vi "weight_experimental2.vi"(9 "IIR Filter Cluster":T1={"filter structure"=enum."IIR 2nd Order", "Reverse Coefficients"=[-0.8648355985677569, 0.0, -1.8688121229267716, 0.9029397901016704, -1.8196275590015545, 0.847351865339388, -1.7873550514945042, 0.8113653291402647, -1.7646245178602125, 0.7862391997716377, -1.7486001722944886, 0.7686314023380645, -1.7316927626267011, 0.7501448296370037, -1.737874982086305, 0.7568937398228854], "Forward Coefficients"=[0.0742867069172382, 0.0742867069172382, 0.0, 0.005985276674302437, 0.011970553348604874, 0.005985276674302437, 0.00581901644640044, 0.01163803289280088, 0.00581901644640044, 0.005710698277145051, 0.011421396554290102, 0.005710698277145051, 0.005634756015992636, 0.011269512031985273, 0.005634756015992636, 0.005581386206513606, 0.011162772413027213, 0.005581386206513606, 0.0055252205885281845, 0.011050441177056369, 0.0055252205885281845, 0.00554574059897006, 0.01109148119794012, 0.00554574059897006]}, 10 "N_points":i32=4200, 11 "PV weight":dbl caption="g" format="%#.0f") -> (1 "Q3":dbl caption="mg/s" format="%#.0f", 2 "Q 1":dbl caption="mg/s" format="%#.0f", 3 "Weight 1":dbl caption="g" format="%#.0f", 5 "This VI":refnum<vi>)   [LabVIEW 2019]
uses:
  <vilib>/Analysis/baseanly.llb/Mean (DBL).vi
  <vilib>/Analysis/baseanly.llb/IIR Cascade Filter (DBL).vi
  <vilib>/Analysis/NI_AALBase.lvlib
panel:
  in  "Tab Control":T2(tab)
  out "dM 3":dbl caption="g" format="%#.0f"
  out "dM 1":dbl caption="g" format="%#.0f"
  out "variance":dbl format="%0.2f"
  out "standard deviation":dbl format="%0.2f"
  in  "Tare":dbl caption="g" format="%#.0f"
  in  "<0>":bool
  in  "<вес>":bool
  in  "k":dbl=1.0 caption="g" format="%#.3f"
  in  "Вес":dbl caption="g" format="%#.0f"
  # "Усреднение за 1 мин"
  # "(расход)"
  # "Усреднение за 3 мин"
  # "(расход)"
  # "Вес тары\n(полностью очистить бункер от продукта\nи запомнить PV weight или ввести вручную)."
  # "Вес тары\n(ввести фактический вес без учета тары\nили ввести k вручную)"
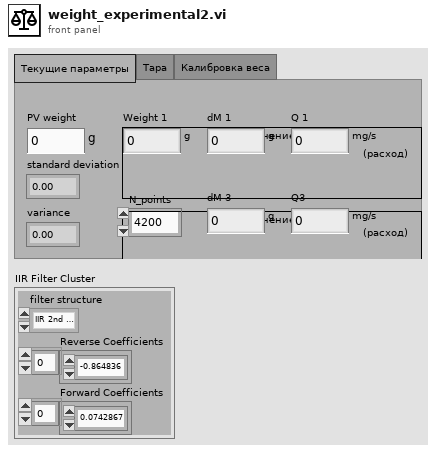
[diagram p1: front panel]
types:
  T1 = cluster{"filter structure":enum32{"IIR 2nd Order", "IIR 4th Order"}, "Reverse Coefficients":dbl[], "Forward Coefficients":dbl[]}
  T2 = enum32{"Текущие параметры", "Тара", "Калибровка веса"}
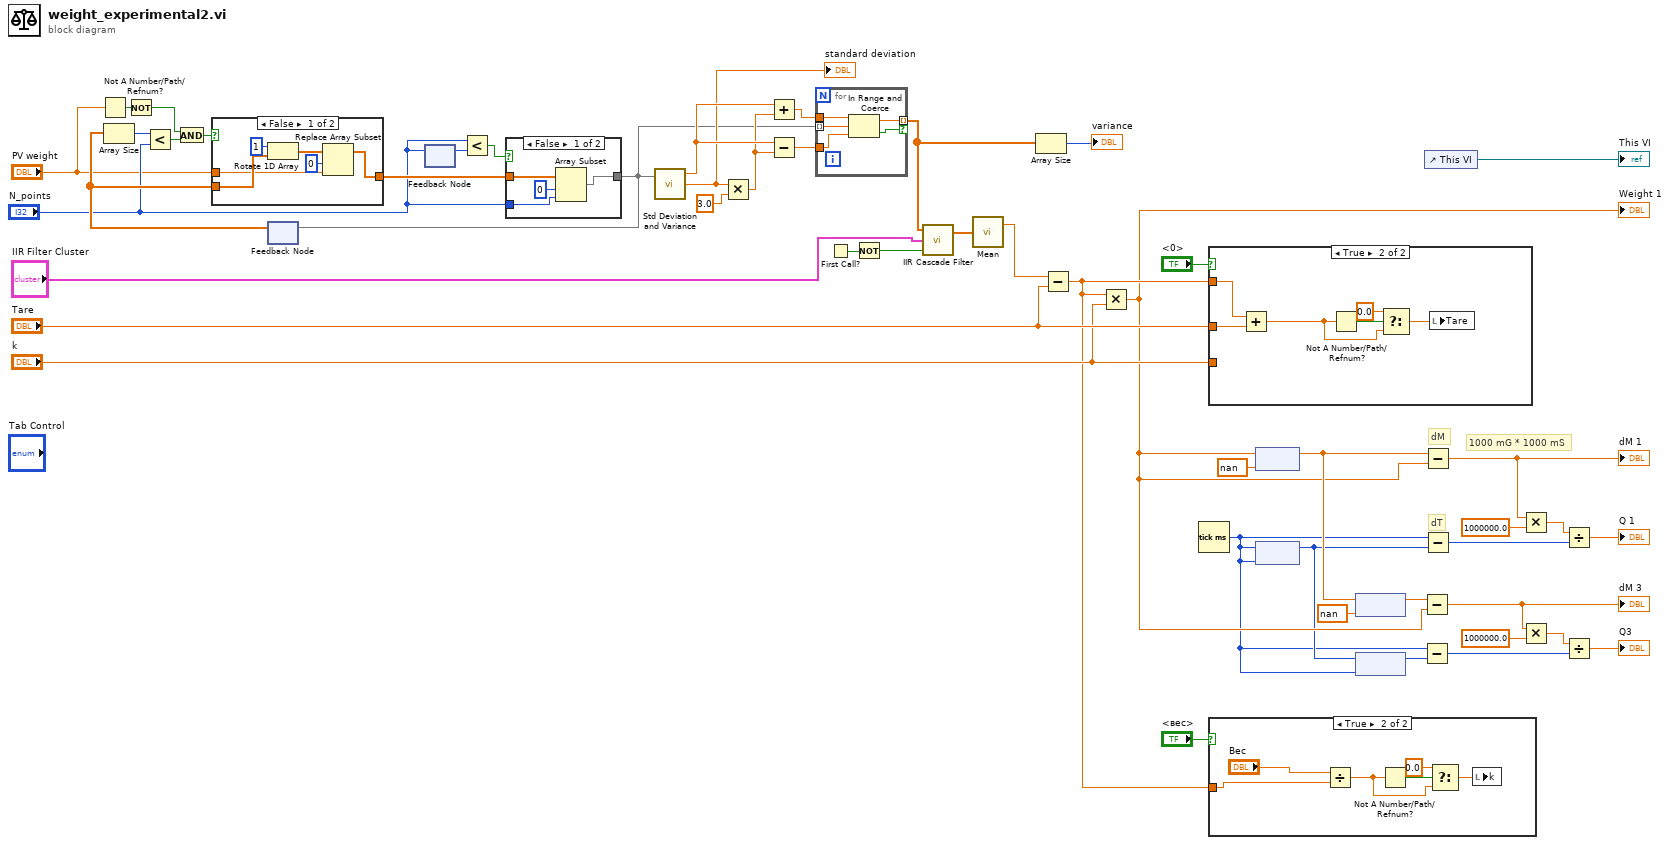
[diagram p0: block diagram]
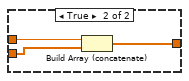
[diagram p3: hidden frame]
diagram:
  # "1000 mG * 1000 mS"
  # "dM"
  # "dT"
  n1 = Not A Number/Path/Refnum?(number/path/refnum="PV weight") -> (NaN/Path/Refnum?=w14:bool)
  n2 = Not(x=w14) -> (.not. x?=w13:bool)
  n3 = feedback #1() -> (w17:dbl[])  [unwired: 1 in]
  n4 = Array Size(array=w17) -> (size(s)=w18:i32)
  n5 = Less?(x=w18, y="N_points") -> (x < y?=w16:bool)
  n6 = And(x=w13, y=w16) -> (x .and. y?=w15:bool)
  n7 = case shown="False" w15 {
    tunnel: [w50 w57] -> w12
    tunnel: "PV weight" -> [w51 w58]
    tunnel: w17 -> [w52 w56]
    frame False {
      n8 = Rotate 1D Array(1:w52, 2:1 ("n")) -> (0:w54:dbl[])
      n9 = Replace Array Subset(array=w54, new element=w51, index=0) -> (w50:dbl[])
    }
    frame True {
      n10 = Build Array (concatenate)(w58, w56) -> (w57:dbl[])
    }
  }
  n11 = feedback #2() -> (w10:i32)  [unwired: 1 in]
  n12 = feedback-in #2("N_points") -> ()
  n13 = Less?(x="N_points", y=w10) -> (x < y?=w9:bool)
  n14 = case shown="False" w9 {
    tunnel: [w61 w63] -> w8
    tunnel: w12 -> [w62 w63]
    tunnel: "N_points" -> [w59 _]
    frame False {
      n15 = Array Subset(array=w62, index=0, length=w59) -> (w61:dbl[])
    }
    frame True {
    }
  }
  n16 = feedback-in #1(w8) -> ()
  n17 = call <vilib>:"Std Deviation and Variance.vi"("X"=w8) -> ("mean"=w25:dbl, "standard deviation"=w21:dbl)  [unwired: 1 in, 1 out]
  "standard deviation" <- w21
  n18 = Multiply(x=w21, y=3.0) -> (x*y=w19:dbl)
  n19 = Add(x=w25, y=w19) -> (x+y=w24:dbl)
  n20 = Subtract(x=w25, y=w19) -> (x-y=w23:dbl)
  n21 = for {
    tunnel: w8 -> [w66] mode=indexing
    tunnel: w24 -> [w68]
    tunnel: w23 -> [w67]
    tunnel: [w65] -> w3 mode=indexing if=w64
    n22 = In Range and Coerce(upper limit=w68, x=w66, lower limit=w67) -> (coerced(x)=w65:dbl, In Range?=w64:bool)
  }
  n23 = First Call?() -> (First Call?: T/F=w7:bool)
  n24 = Not(x=w7) -> (.not. x?=w6:bool)
  n25 = call-poly <vilib>:"IIR Cascade Filter.vi"("init/cont (init:F)"=w6, "IIR Filter Cluster"="IIR Filter Cluster", "X"=w3) -> ("Filtered X"=w2:dbl[])  [unwired: 1 out]
  n26 = call-poly <vilib>:"Mean.vi"("X"=w2) -> ("mean"=w1:dbl)  [unwired: 1 out]
  n27 = Array Size(array=w3) -> (size(s)=→"variance":i32)
  n28 = Subtract(x=w1, y="Tare") -> (x-y=w36:dbl)
  n29 = Multiply(x=w36, y="k") -> (x*y=w34:dbl)
  "Weight 1" <- w34
  n30 = Tick Count (ms)() -> (millisecond timer value=w31:u32)
  n31 = case shown="True" "<0>" {
    tunnel: "Tare" -> [_ w71]
    tunnel: w36 -> [_ w70]
    tunnel: "k" -> [_ _]
    frame False {
    }
    frame True {
      n32 = Add(x=w70, y=w71) -> (x+y=w69:dbl)
      n33 = Not A Number/Path/Refnum?(number/path/refnum=w69) -> (NaN/Path/Refnum?=w74:bool)
      n34 = Select(t=0.0 ("y"), s=w74, f=w69) -> (s? t:f=w72:dbl)
      n35 = local write "Tare"(w72) -> ()
    }
  }
  n36 = case shown="True" "<вес>" {
    tunnel: w36 -> [_ w75]
    frame False {
    }
    frame True {
      n37 = Divide(x="Вес", y=w75) -> (x/y=w78:dbl)
      n38 = Not A Number/Path/Refnum?(number/path/refnum=w78) -> (NaN/Path/Refnum?=w80:bool)
      n39 = Select(t=0.0 ("y"), s=w80, f=w78) -> (s? t:f=w77:dbl)
      n40 = local write "k"(w77) -> ()
    }
  }
  n41 = feedback #3(nan) -> (w45:dbl)
  n42 = feedback-in #3(w34) -> ()
  n43 = feedback #4(w31) -> (w33:u32)
  n44 = feedback-in #4(w31) -> ()
  n45 = feedback #5(nan) -> (w46:dbl)
  n46 = feedback-in #5(w45) -> ()
  n47 = feedback #6(w31) -> (w32:u32)
  n48 = feedback-in #6(w33) -> ()
  n49 = Subtract(x=w46, y=w34) -> (x-y=w27:dbl)
  "dM 3" <- w27
  n50 = Subtract(x=w31, y=w32) -> (x-y=w28:u32)
  n51 = Subtract(x=w45, y=w34) -> (x-y=w40:dbl)
  "dM 1" <- w40
  n52 = Subtract(x=w31, y=w33) -> (x-y=w38:u32)
  n53 = control-ref of="This VI"() -> (→"This VI":refnum<vi>)
  n54 = Multiply(x=w40, y=1000000.0) -> (x*y=w39:dbl)
  n55 = Multiply(x=w27, y=1000000.0) -> (x*y=w30:dbl)
  n56 = Divide(x=w39, y=w38) -> (x/y=→"Q 1":dbl)
  n57 = Divide(x=w30, y=w28) -> (x/y=→"Q3":dbl)
